vi "getFunctionBlocks.vi"(8 "error in (no error)":errorcluster, 11 "IFunctionBlock in":refnum<class "IFunctionBlock.lvclass">) -> (0 "error out":errorcluster, 2 "IFunctionBlocks out":refnum<class "IFunctionBlock.lvclass">[](array[class]), 3 "IFunctionBlock out":refnum<class "IFunctionBlock.lvclass">)   [LabVIEW 2022 SP3, in "openDAQ.lvlib" / "IBaseObject.lvlib" / "IPropertyObject.lvlib" / "IComponent.lvlib" / "IFolder.lvlib" / "IFunctionBlock.lvlib" / "IFunctionBlock.lvclass"]
uses:
  <instrlib>/openDAQ/Public/Classes/IFunctionBlock/IFunctionBlock.lvclass
  <instrlib>/openDAQ/Public/Classes/IFunctionBlock/IFunctionBlock.lvclass/IFunctionBlock.ctl
  <instrlib>/openDAQ/Public/Classes/daqCoreTypes/IList/IList.lvclass
  <instrlib>/openDAQ/Public/Classes/daqCoreTypes/IList/Polymorphic/getList/getFunctionBlockList.vi
  <instrlib>/openDAQ/Binaries/Windows/x86/copendaq32.dll
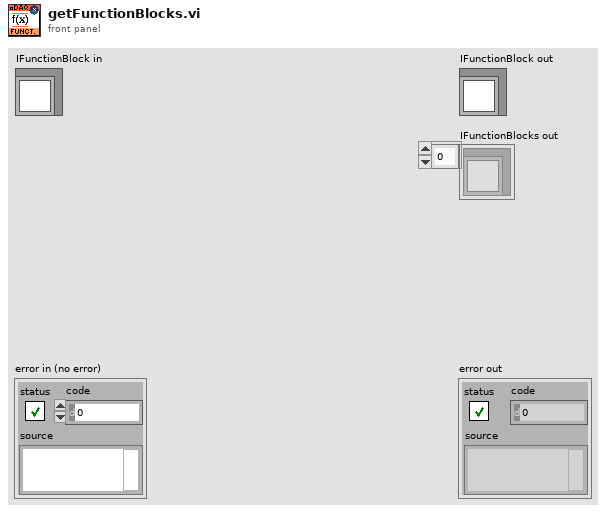
[diagram p1: front panel]
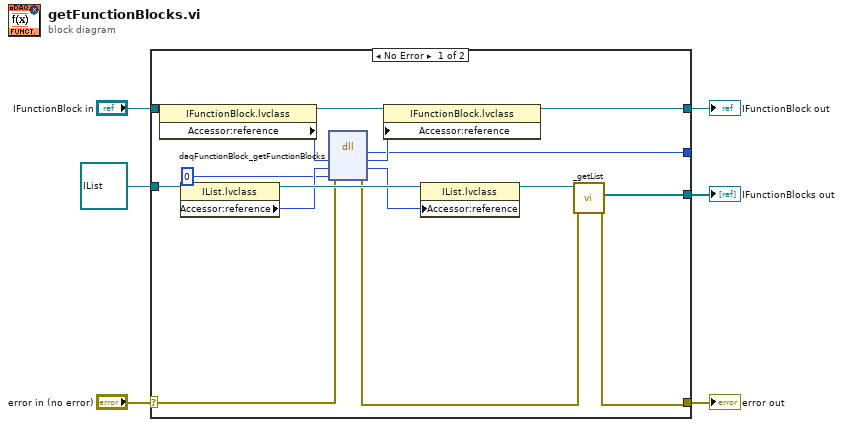
[diagram p0: block diagram]
diagram:
  n1 = case shown="No Error" "error in (no error)" {
    selector: "error in (no error)" -> [w13 w24]
    tunnel: [w9 w24] -> w5
    tunnel: [w20 w23] -> w3
    tunnel: "IFunctionBlock in" -> [w21 w23]
    tunnel: refnum<class "IList.lvclass"> refnum ("openDAQ.lvlib:daqCoreTypes.lvlib:IList.lvclass") -> [w16 _]
    tunnel: [w11 _] -> w1
    tunnel: [w7 _] -> _
    frame No Error {
      n2 = property class="IFunctionBlock.lvclass"(reference=w21) -> (reference out=w19:refnum<class "IFunctionBlock.lvclass">, "Accessor:reference"=w18:i64)  [unwired: 1 in, 1 out]
      n3 = property class="IList.lvclass"(reference=w16) -> (reference out=w22:refnum<class "IList.lvclass">, "Accessor:reference"=w15:i64)  [unwired: 1 in, 1 out]
      n4 = dll-call lib="C:/Program Files (x86)/National Instruments/LabVIEW 2022/instr.lib/openDAQ/Binaries/Windows/x86/copendaq*.*" fn="daqFunctionBlock_getFunctionBlocks"(error in=w13, "functionBlock"=w18, "functionBlocks"=w15, "searchFilter"=i64 0) -> (error out=w10:errorcluster, "return type"=w7:u32, "functionBlock"=w17:i64, "functionBlocks"=w14:i64)  [unwired: 3 in, 1 out]
      n5 = property class="IFunctionBlock.lvclass"(reference=w19, "Accessor:reference"=w17) -> (reference out=w20:refnum<class "IFunctionBlock.lvclass">)  [unwired: 1 in, 1 out]
      n6 = property class="IList.lvclass"(reference=w22, "Accessor:reference"=w14) -> (reference out=w12:refnum<class "IList.lvclass">)  [unwired: 1 in, 1 out]
      n7 = call-poly <instrlib>:"_getList.vi"("error in (no error)"=w10, "IList in"=w12) -> ("error out"=w9:errorcluster, "devices out"=w11:refnum<class "IFunctionBlock.lvclass">[])  [unwired: 8 in]
    }
    frame Error {
    }
  }
  "error out" <- w5
  "IFunctionBlock out" <- w3
  "IFunctionBlocks out" <- w1
